vi "getInstanceTcpServer.vi"(8 "error in (no error)":errorcluster, 11 "tcpServer in":refnum<class "TcpServer.lvclass">) -> (0 "error out":errorcluster, 1 "TcpServer":refnum<user-event>, 2 "TcpServer":refnum<user-event>, 3 "tcpServer out":refnum<class "TcpServer.lvclass">)   [LabVIEW 2018, in "TcpServer.lvclass"]
doc: "Get the TCP Server user event instance. There are two TcpServer user event references: one for TcpServerCmd and one for TcpServerTel."
uses:
  TcpServer.lvclass
  TcpServer.lvclass/TcpServer.ctl
  TcpServerBase/TcpServerBase.lvclass/TcpServerBase.ctl
  TcpServerCmd/TcpServerCmd.lvclass
  home/pcortes/github/ts_labview_tcp_json/src/TcpServerBase/TcpServerBase.lvclass
  TcpServerTel/TcpServerTel.lvclass
  TcpServerBase/TcpServerBase.lvclass
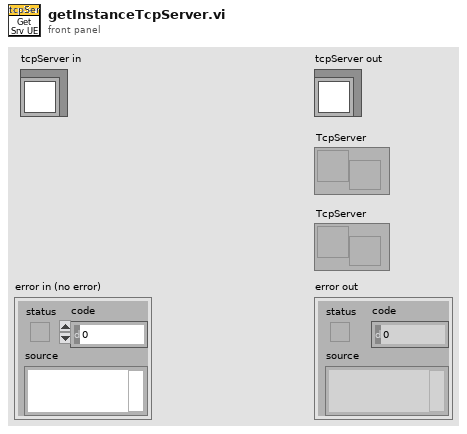
[diagram p1: front panel]
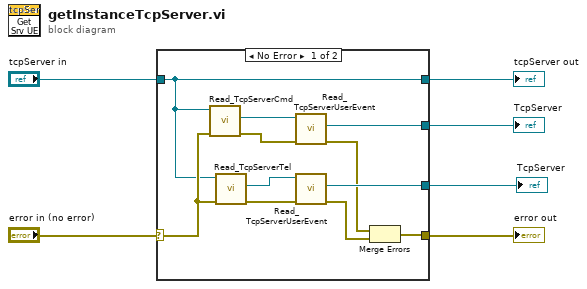
[diagram p0: block diagram]
diagram:
  n1 = case shown="No Error" "error in (no error)" {
    selector: "error in (no error)" -> [w14 w19]
    tunnel: [w9 w19] -> w5
    tunnel: [w11 w18] -> w2
    tunnel: "tcpServer in" -> [w11 w18]
    tunnel: [w17 _] -> w3
    tunnel: [w10 _] -> w1
    frame No Error {
      n2 = call "Read_TcpServerCmd.vi"("error in (no error)"=w14, "TcpServer in"=w11) -> ("error out"=w15:errorcluster, "TcpServerCmd.lvclass"=w16:refnum<class "TcpServerCmd.lvclass">)  [unwired: 7 in, 1 out]
      n3 = call "Read_TcpServerTel.vi"("error in (no error)"=w14, "TcpServer in"=w11) -> ("error out"=w12:errorcluster, "TcpServerTel.lvclass"=w13:refnum<class "TcpServerTel.lvclass">)  [unwired: 7 in, 1 out]
      n4 = call "Read_TcpServerUserEvent.vi"("error in (no error)"=w15, "TcpServerBase in"=w16) -> ("error out"=w8:errorcluster, "TcpServer"=w17:refnum<user-event>)  [unwired: 7 in, 1 out]
      n5 = call "Read_TcpServerUserEvent.vi"("error in (no error)"=w12, "TcpServerBase in"=w13) -> ("error out"=w7:errorcluster, "TcpServer"=w10:refnum<user-event>)  [unwired: 7 in, 1 out]
      n6 = Merge Errors(w8, w7) -> (w9:errorcluster)
    }
    frame Error {
    }
  }
  "error out" <- w5
  "tcpServer out" <- w2
  "TcpServer" <- w3
  "TcpServer" <- w1
